vi "GUNSC_inspectErros.vi"(6 "show Dialog?":bool, 7 "message":string, 8 "error in (no error)":errorcluster, 10 "errostr":string, 11 "error code":i32) -> (0 "error out":errorcluster)   [LabVIEW 2014]
doc: "This subVI tests the error status output of one or more low-level functions or subVIs that output a numeric error code, and creates an error out cluster that can be wired to the Simple or General Error Handler in order to identify the error and describe it to the user.\n\nThe error in cluster is tested first. If error? is no-error, the elements of the error codes array are tested next for non-zero values. The first error found terminates the test, and error out identifies that error. Use a Build Array function to assemble the individual error codes.\n\nYou can optionally use the source messages string to pass on the source of the error. Enter one line of text for each element of the error codes array. \n\nThe error? status is TRUE on any error."
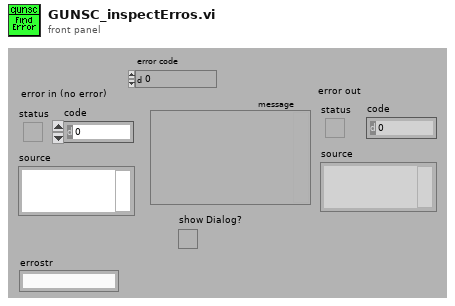
[diagram p1: front panel]
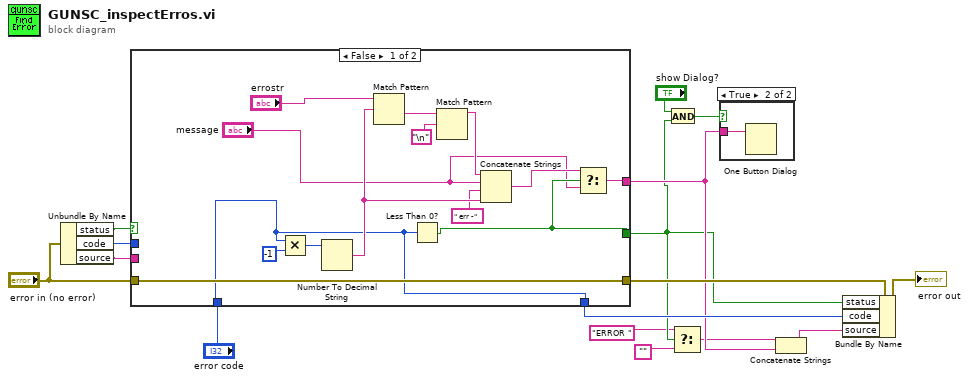
[diagram p0: block diagram]
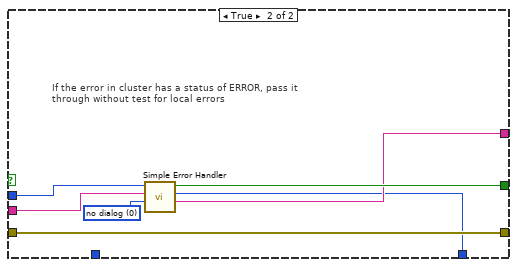
[diagram p3: hidden frame]
diagram:
  n1 = Unbundle By Name("error in (no error)") -> ("status"=w12:bool, "code"=w13:i32, "source"=w11:string)
  n2 = case shown="False" w12 {
    tunnel: "error in (no error)" -> [w30 w37]
    tunnel: [w30 w37] -> w10
    tunnel: [w21 w34] -> w6
    tunnel: [w19 w35] -> w4
    tunnel: w13 -> [_ w33]
    tunnel: w11 -> [_ w36]
    tunnel: "error code" -> [w20 _]
    tunnel: [w20 w32] -> w7
    frame False {
      n3 = Multiply(x=w20, y=-1) -> (x*y=w23:i32)
      n4 = Number To Decimal String(number=w23) -> (decimal integer string=w26:string)  [unwired: 1 out]
      n5 = Match Pattern(string="errostr", regular expression=w26) -> (after substring=w28:string)  [unwired: 4 out]
      n6 = Less Than 0?(x=w20) -> (x < 0?=w19:bool)
      n7 = Match Pattern(string=w28, regular expression="\n") -> (before substring=w24:string)  [unwired: 4 out]
      n8 = Concatenate Strings(w24, "message", " err -", w26) -> (w22:string)
      n9 = Select(t=w22, s=w19, f="message") -> (s? t:f=w21:string)
    }
    frame True {
      w31 = u16 0 items=["no dialog", "OK message", "continue or stop message"] ("type of dialog (OK msg:1)")
      # "If the error in cluster has a status of ERROR, pass it through without test for local errors"
      n10 = call <vilib>:"Simple Error Handler.vi"("error code (no error:0)"=w33, "error source (\" \")"=w36, "type of dialog (OK msg:1)"=w31) -> ("error?"=w35:bool, "code out"=w32:i32, "source out"=w34:string)  [unwired: 1 in, 3 out]
    }
  }
  n11 = And(x="show Dialog?", y=w4) -> (x .and. y?=w14:bool)
  n12 = Select(t="ERROR ", s=w4, f="") -> (s? t:f=w1:string)
  n13 = case shown="True" w14 {
    tunnel: w6 -> [_ w38]
    frame False {
    }
    frame True {
      n14 = One Button Dialog(message=w38) -> ()  [unwired: 2 out]
    }
  }
  n15 = Concatenate Strings(w1, w6) -> (w5:string)
  n16 = Bundle By Name(cluster=w10, "status"=w4, "code"=w7, "source"=w5) -> (→"error out":errorcluster)
